vi "Send_Test_Email.vi"() -> ()   [LabVIEW 2010]
uses:
  Anemometry Sub Vis/Controls/Post_Process.ctl
  Anemometry Sub Vis/Globals/Meas_global.vi
  Anemometry Sub Vis/Utilities/Email_transfer_global.vi
panel:
  in  "Extra People to Email":string[](array[string])=["p.hayden@surrey.ac.uk"]
  in  "Message":string
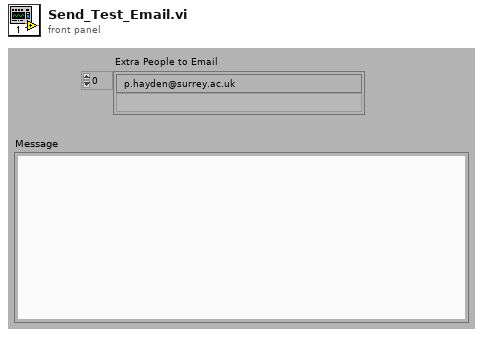
[diagram p1: front panel]
types:
  T1 = typedef "Post_Process.ctl" = enum16{"Take New Data", "Post Process Raw Data File"}
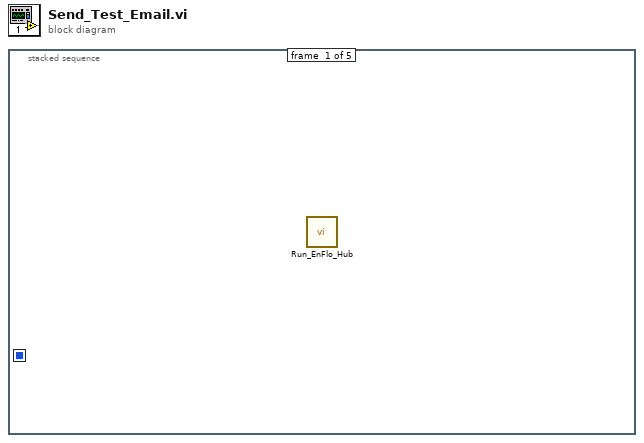
[diagram p0: block diagram]
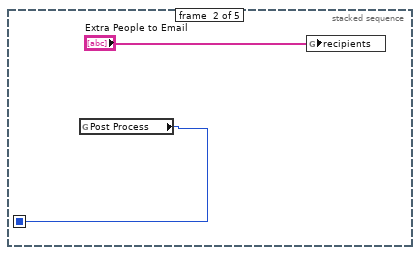
[diagram p2: hidden frame]
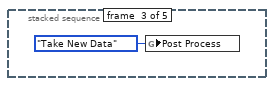
[diagram p3: hidden frame]
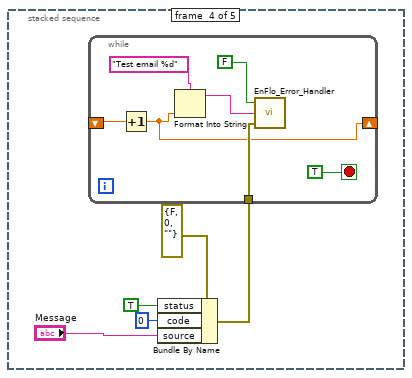
[diagram p4: hidden frame]
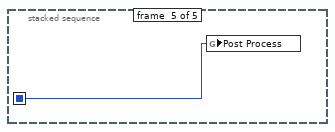
[diagram p5: hidden frame]
diagram:
  n1 = stacked-sequence {
    seq-local: [_ w1 _ _ _] -> [_ _ _ _ w16]
    frame #0 {
      n2 = call "Run_EnFlo_Hub.vi"() -> ()  [unwired: 8 out]
    }
    frame #1 {
      n3 = global read "Meas_global.vi" "Post Process"() -> (w1:T1)
      n4 = global write "Email_transfer_global.vi" "recipients"("Extra People to Email") -> ()
    }
    frame #2 {
      n5 = global write "Meas_global.vi" "Post Process"(Post_Process."Take New Data" ("Post Process")) -> ()
    }
    frame #3 {
      n6 = Bundle By Name(cluster=errorcluster {"status"=FALSE, "code"=0, "source"=""} ("error in (no error)"), "status"=TRUE, "code"=0, "source"="Message") -> (w7:errorcluster)
      n7 = while {
        tunnel: w7 -> [w14]
        shift-right: [w9] -> _
        shift-left: _ -> [w10]
        stop <- TRUE stop-if-true
        n8 = Increment(x=w10) -> (x+1=w9:dbl)
        n9 = Format Into String(format string="Test email %d" ("Error Type"), w9) -> (resulting string=w12:string)  [unwired: 2 in, 1 out]
        n10 = call "EnFlo_Error_Handler.vi"("error in (no error)"=w14, "Error Type"=w12, "Dialog Box (T)"=FALSE) -> ()  [unwired: 3 out]
      }
    }
    frame #4 {
      n11 = global write "Meas_global.vi" "Post Process"(w16) -> ()
    }
  }
